vi "ExitVI.vi"(8 "error in (no error)":errorcluster) -> (0 "error out (no error)":errorcluster)   [LabVIEW 2020]
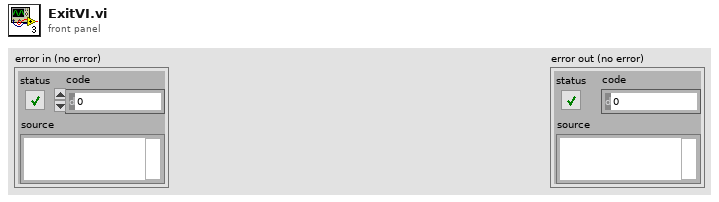
[diagram p1: front panel]
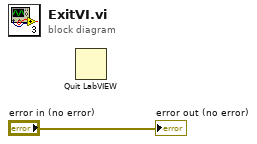
[diagram p0: block diagram]
diagram:
  n1 = Quit LabVIEW() -> ()  [unwired: 1 in]
  "error out (no error)" <- "error in (no error)"
